vi "Get Routing Channel.vi"(8 "error in (no error)":errorcluster, 11 "Channel Ref in":T1 format="%.0x") -> (0 "error out":errorcluster, 1 "Channel States":T2, 2 "Channel Name":string, 3 "Channel Ref out":T1 format="%.0x", 4 "Description":string)   [LabVIEW 2017, in "Switch Scripting.lvlib"]
uses:
  Switch Scripting.lvlib
  <vilib>/NI Veristand/Custom Device API/Custom Device Item Ref.ctl
  Channel States.ctl
  Routing State.ctl
  Connection.ctl
  <vilib>/NI VeriStand/Custom Device API/Custom Device API.lvlib
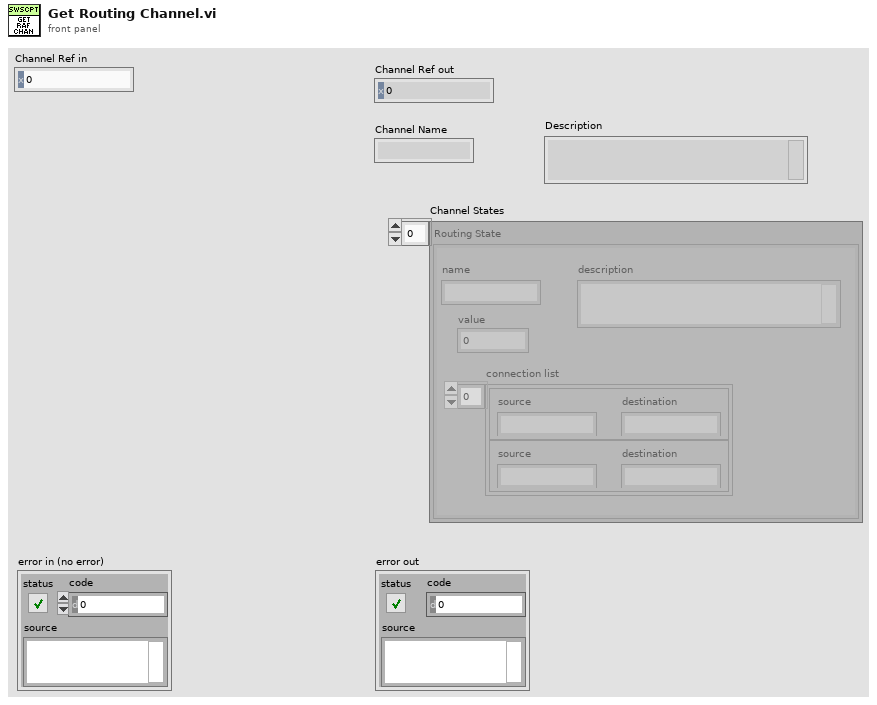
[diagram p1: front panel]
types:
  T1 = typedef "Custom Device API.lvlib/Custom Device Item Ref.ctl" = u64
  T2 = typedef "Switch Scripting.lvlib/Channel States.ctl" = T3[]
  T3 = typedef "Switch Scripting.lvlib/Routing State.ctl" = cluster{"name":string, "description":string, "value":i32, "connection list":T4[]}
  T4 = typedef "Switch Scripting.lvlib/Connection.ctl" = cluster{"source":string, "destination":string}
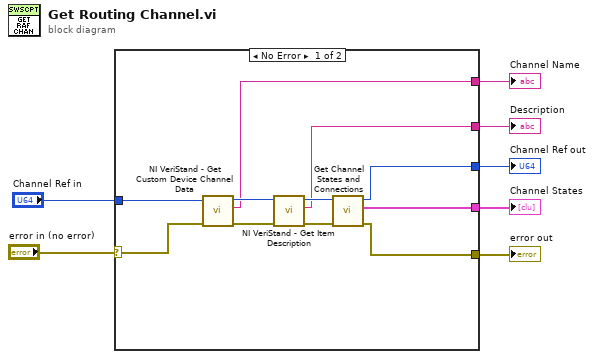
[diagram p0: block diagram]
diagram:
  n1 = case shown="No Error" "error in (no error)" {
    selector: "error in (no error)" -> [w18 w19]
    tunnel: [w16 w19] -> w7
    tunnel: "Channel Ref in" -> [w15 _]
    tunnel: [w9 _] -> w3
    tunnel: [w17 _] -> w4
    tunnel: [w14 _] -> w2
    tunnel: [w8 _] -> w1
    frame No Error {
      n2 = call <vilib>:"NI VeriStand - Get Custom Device Channel Data.vi"("error in (no error)"=w18, "Channel Ref in"=w15) -> ("error out"=w11:errorcluster, "Channel Name"=w9:string, "Channel Ref out"=w13:T1)  [unwired: 4 in, 3 out]
      n3 = call <vilib>:"NI VeriStand - Get Item Description.vi"("error in (no error)"=w11, "Item Ref in"=w13) -> ("error out"=w10:errorcluster, "Description"=w8:string, "Item Ref out"=w12:T1)  [unwired: 6 in, 1 out]
      n4 = call "Get Channel States and Connections.vi"("error in (no error)"=w10, "Channel Ref in"=w12) -> ("error out"=w16:errorcluster, "Routing Channel States"=w17:T2, "Channel Ref out"=w14:T1)  [unwired: 7 in]
    }
    frame Error {
    }
  }
  "error out" <- w7
  "Channel Name" <- w3
  "Channel States" <- w4
  "Channel Ref out" <- w2
  "Description" <- w1
